vi "Get Identifier.vi"(8 "Error In":errorcluster, 11 "reference in":refnum<class "NI9862.lvclass">) -> (0 "Error Out":errorcluster, 2 "Identifier":string, 3 "reference out":refnum<class "NI9862.lvclass">)   [LabVIEW 2024, in "NI9862.lvclass"]
uses:
  NI9862.lvclass
  NI9862.lvclass/NI9862.ctl
  Source/Interfaces/IInstrument/IInstrument.lvclass
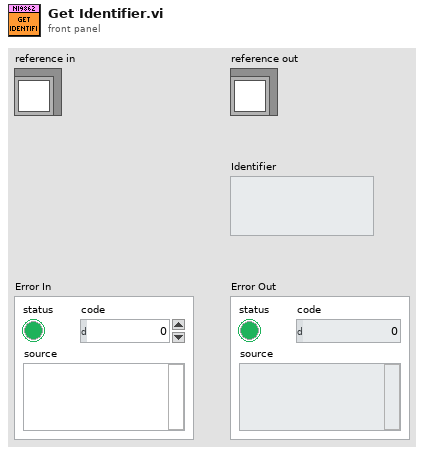
[diagram p1: front panel]
types:
  T1 = typedef "NI9862.lvclass/ObjectAttributes.ctl" = cluster{"IConfigure":refnum<class "IConfigure.lvclass">}
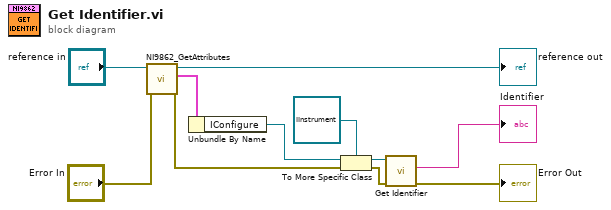
[diagram p0: block diagram]
diagram:
  n1 = call "NI9862_GetAttributes.vi"("Error In"="Error In", "NI9862 in"="reference in") -> ("Error Out"=w2:errorcluster, "Data"=w6:T1, "NI9862 out"=→"reference out":refnum<class "NI9862.lvclass">)  [unwired: 6 in, 1 out]
  n2 = Unbundle By Name(w6) -> ("IConfigure"=w5:refnum<class "IConfigure.lvclass">)
  n3 = To More Specific Class(target class=refnum<class "IInstrument.lvclass"> refnum ("IInstrument.lvclass"), reference=w5, error in=w2) -> (specific class reference=w4:refnum<class "IInstrument.lvclass">, error out=w1:errorcluster)
  n4 = call-dynamic "Get Identifier.vi"("error in"=w1, "IInstrument in"=w4) -> ("error out"=→"Error Out":errorcluster, "Identifier"=→"Identifier":string)  [unwired: 7 in, 1 out]
